vi "Dispose Kinect.vi"(4 "error in (no error)":errorcluster, 7 "Reference In":T1) -> (0 "error out":errorcluster)   [LabVIEW 2010]
uses:
  <vilib>/vision/Image Controls.llb/IMAQ Image.ctl
  Microsoft.Research.Kinect
types:
  T1 = cluster{cluster{"queue out":refnum<queue>, "queue out":refnum<queue>}, cluster{"new reference":refnum<k24>, "DepthStream":refnum<k24>, "VideoStream":refnum<k24>, "Event Callback":refnum<k27>, "Event Callback":refnum<k27>}}
  T2 = cluster{"queue out":refnum<queue>, "queue out":refnum<queue>}
  T3 = cluster{"new reference":refnum<k24>, "DepthStream":refnum<k24>, "VideoStream":refnum<k24>, "Event Callback":refnum<k27>, "Event Callback":refnum<k27>}
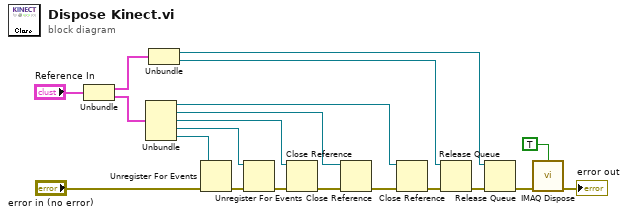
[diagram p0: block diagram]
diagram:
  n1 = Unbundle("Reference In") -> (w1:T2, w2:T3)
  n2 = Unbundle(w2) -> ("new reference"=w16:refnum<k24>, "DepthStream"=w15:refnum<k24>, "VideoStream"=w14:refnum<k24>, "Event Callback"=w13:refnum<k27>, "Event Callback"=w12:refnum<k27>)
  n3 = Unbundle(w1) -> ("queue out"=w7:refnum<queue>, "queue out"=w8:refnum<queue>)
  n4 = Unregister For Events(event registration refnum=w12, error in="error in (no error)") -> (error out=w19:errorcluster)
  n5 = Unregister For Events(event registration refnum=w13, error in=w19) -> (error out=w18:errorcluster)
  n6 = Close Reference(reference=w14, error in (no error)=w18) -> (error out=w20:errorcluster)
  n7 = Close Reference(reference=w15, error in (no error)=w20) -> (error out=w17:errorcluster)
  n8 = Close Reference(reference=w16, error in (no error)=w17) -> (error out=w10:errorcluster)
  n9 = Release Queue(queue=w8, error in (no error)=w10) -> (error out=w9:errorcluster)  [unwired: 1 in, 2 out]
  n10 = Release Queue(queue=w7, error in (no error)=w9) -> (error out=w6:errorcluster)  [unwired: 1 in, 2 out]
  n11 = call "IMAQ Dispose"("All Images? (No)"=TRUE, "error in (no error)"=w6) -> ("error out"=→"error out":errorcluster)  [unwired: 4 in]
